vi "Localization Demo.vi"() -> ()   [LabVIEW 2019]
uses:
  SubVIs/RegisterVI.vi
  <vilib>/Platform/browser.llb/Open URL in Default Browser (string).vi
panel:
  in  "Button with Multiple Strings":bool
  out "Current Date and Time":string caption="Current Date or Time"
  in  "Date and Time":u16(ring) items=["Show Localized Time", "Show Localized Date"]
  in  "Show Dialog":bool caption="Show Localized Dialog"
  in  "Language ListBox":i32(listbox) caption="Language"
  out "Data.Display":dbl(graph) caption="Incoming Data"
  out "Error":bool
  in  "CustomControl.Increment":bool caption="Increment"
  out "Count":dbl
  in  "Exit":bool
  # "Instructions:\n1. Run this VI\n2. Toggle the language selector to show the language you would like to show\n3. Observe that the text on the VI changes language\n4. Push the button that says \"Show Localized Dialog.\" This will call Localize Phrase to show a dialog with a localized phrase.\n5. Check out the github page for more documentation and details\nhttps://github.com/JKISoftware/JKI-Simple-Localization"
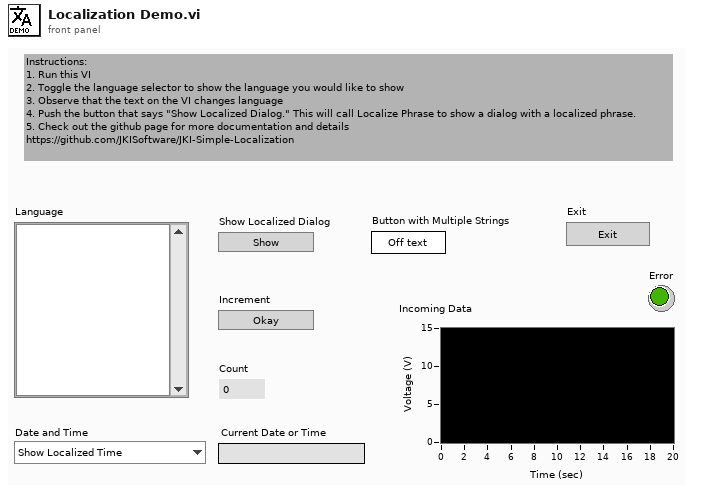
[diagram p1: front panel]
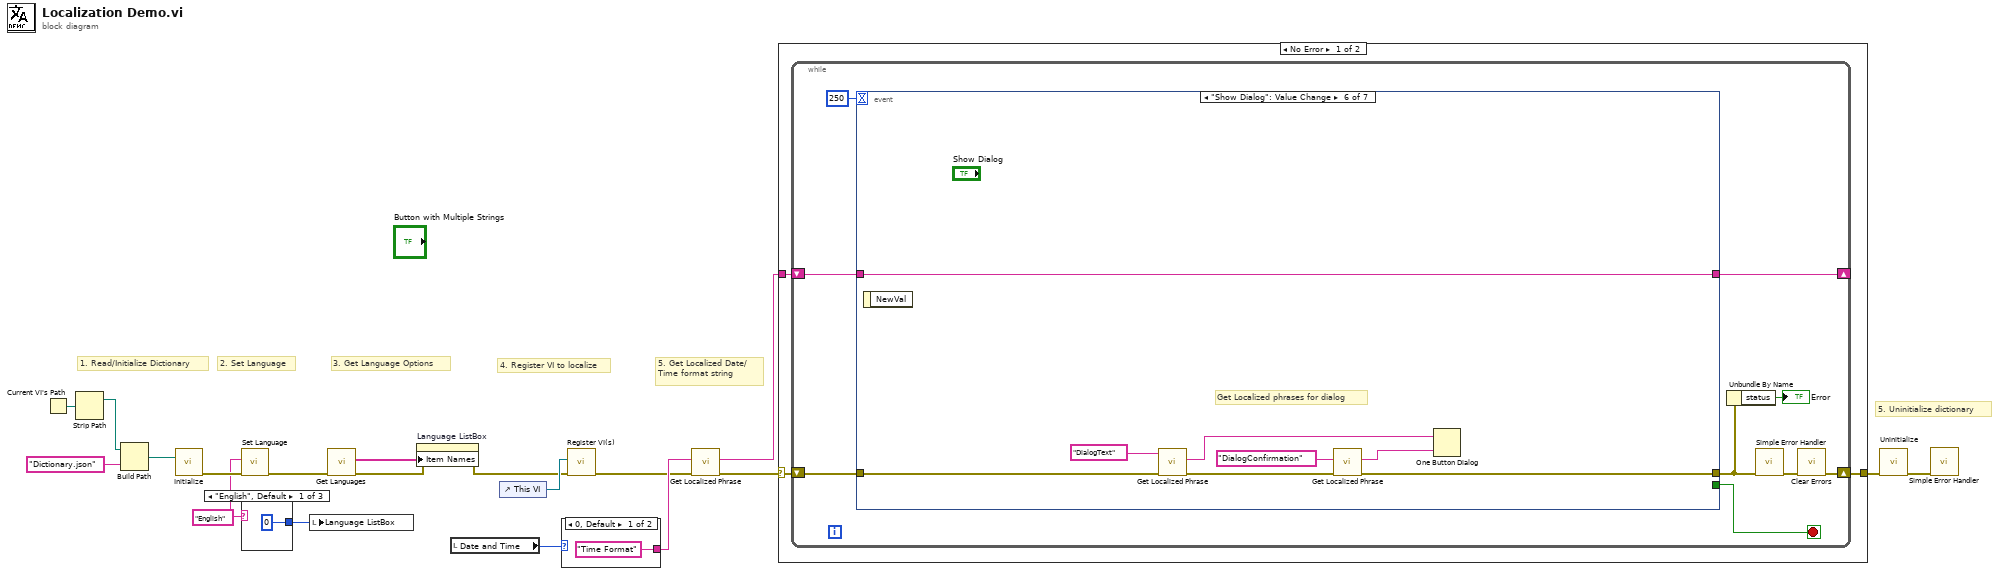
[diagram p0: block diagram]
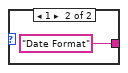
[diagram p2: hidden frame]
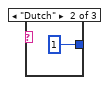
[diagram p3: hidden frame]
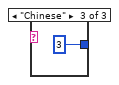
[diagram p4: hidden frame]
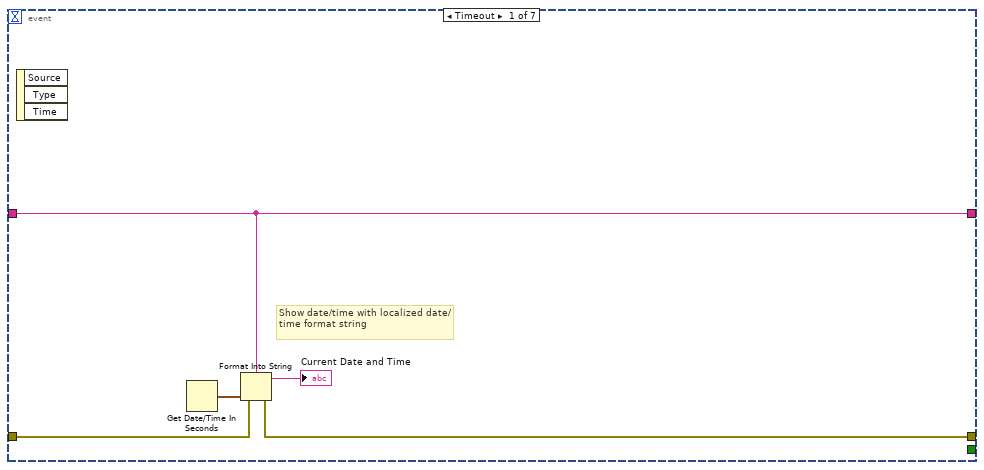
[diagram p5: hidden frame]
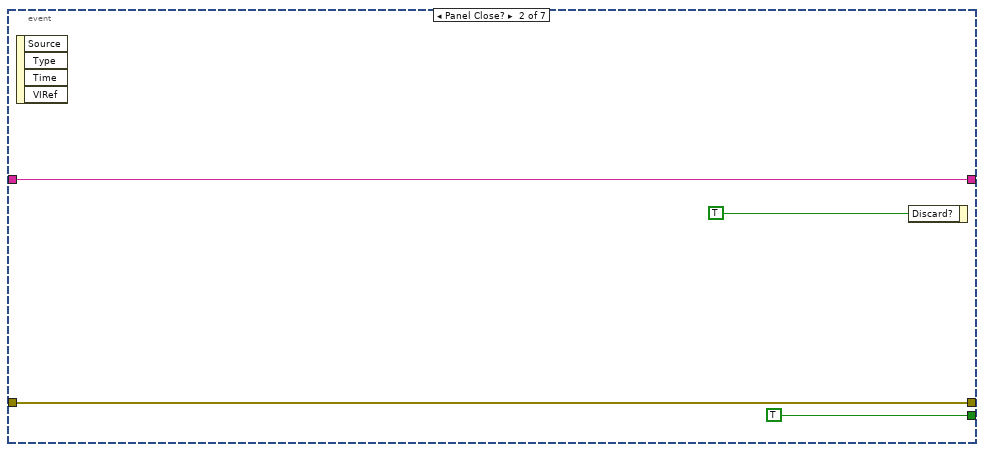
[diagram p6: hidden frame]
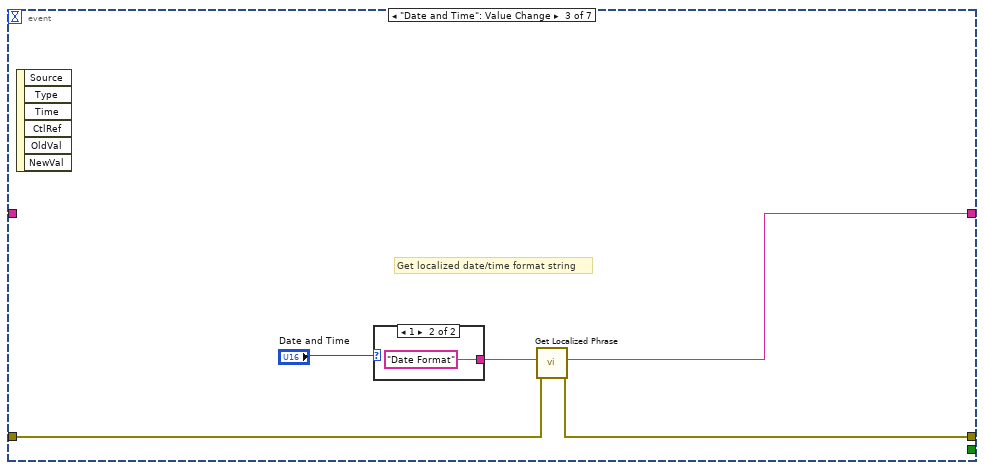
[diagram p7: hidden frame]
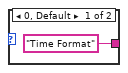
[diagram p8: hidden frame]
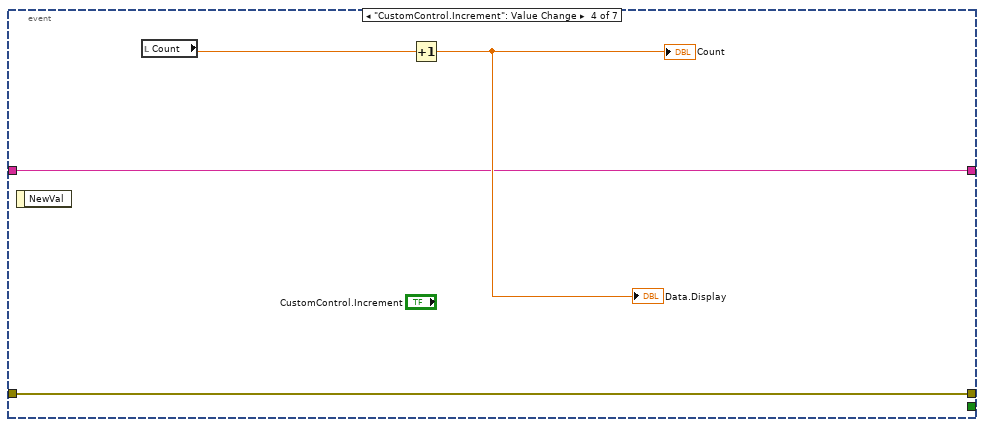
[diagram p9: hidden frame]
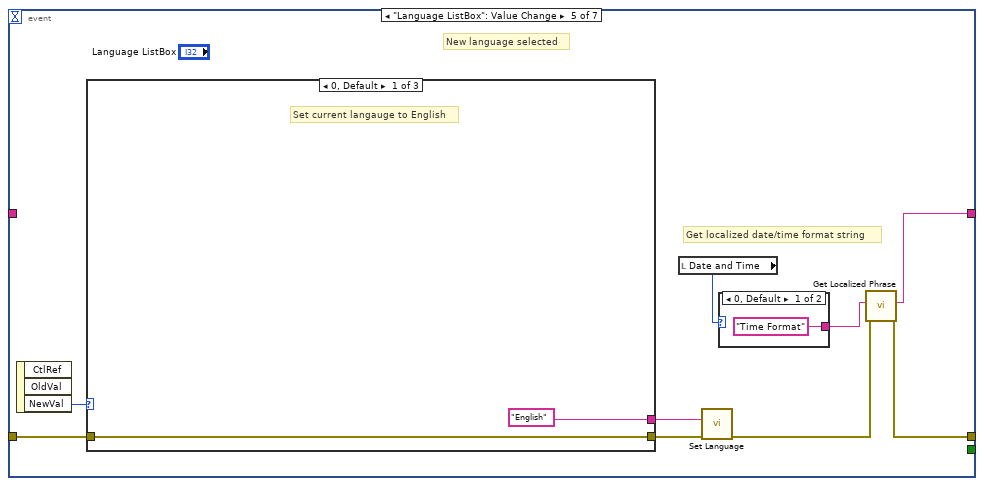
[diagram p10: hidden frame]
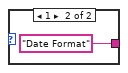
[diagram p11: hidden frame]
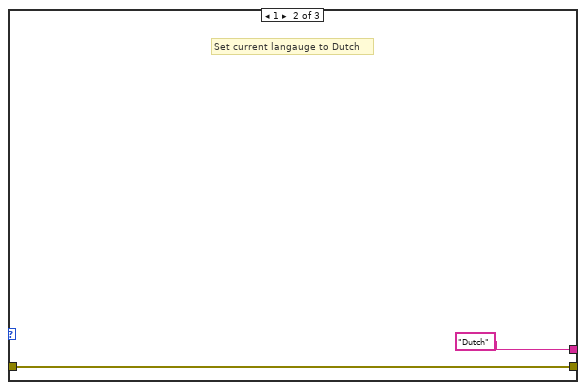
[diagram p12: hidden frame]
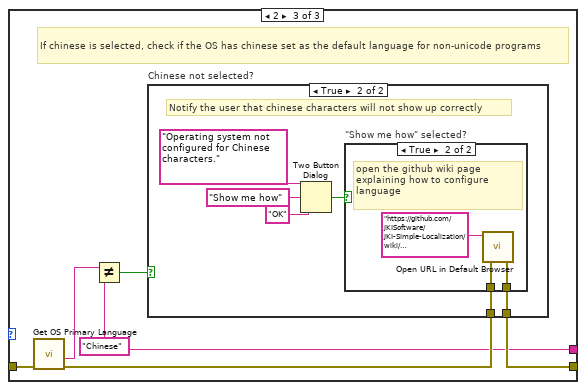
[diagram p13: hidden frame]
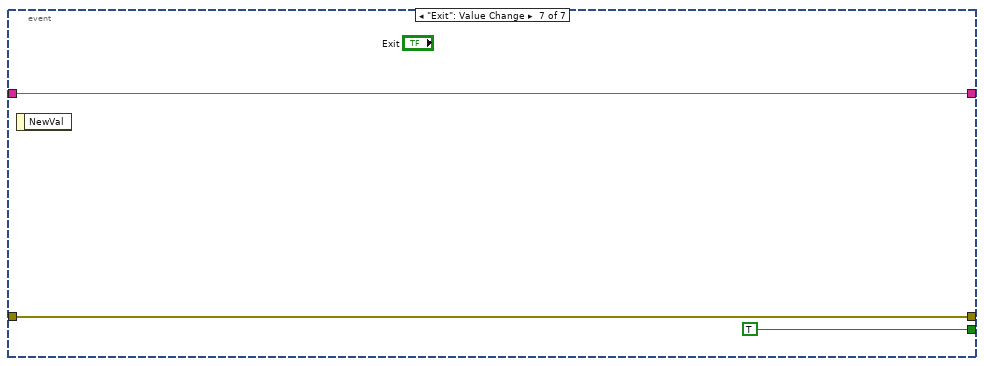
[diagram p16: hidden frame]
diagram:
  w7 = "English" ("Target Language (current lang)")
  # "5. Uninitialize dictionary"
  # "5. Get Localized Date/Time format string"
  # "4. Register VI to localize"
  # "3. Get Language Options"
  # "2. Set Language"
  # "1. Read/Initialize Dictionary"
  n1 = Current VI's Path() -> (path=w11:path)
  n2 = Strip Path(path=w11) -> (stripped path=w10:path)  [unwired: 1 out]
  n3 = Build Path(base path=w10, name or relative path="Dictionary.json") -> (appended path=w19:path)
  n4 = call "Initialize.vi"("Dictionary File Path"=w19) -> ("error out"=w9:errorcluster)  [unwired: 9 in, 5 out]
  n5 = call "Set Language.vi"("error in"=w9, "Target Language (current lang)"=w7) -> ("error out"=w8:errorcluster)  [unwired: 8 in, 1 out]
  n6 = case shown="\"English\", Default" w7 {
    tunnel: [0 ("Language ListBox") 1 ("Language ListBox") 3 ("Language ListBox")] -> w13
    frame "English", Default {
    }
    frame "Dutch" {
    }
    frame "Chinese" {
    }
  }
  n7 = local write "Language ListBox"(w13) -> ()
  n8 = call "Get Languages.vi"("error in"=w8) -> ("error out"=w16:errorcluster, "Languages"=w17:string[])  [unwired: 9 in]
  n9 = property on="Language ListBox" class="LstBox (strict)"(error in=w16, "Item Names"=w17) -> (error out=w14:errorcluster)  [unwired: 1 in, 1 out]
  n10 = local read "Date and Time"() -> (w2:u16)
  n11 = control-ref of="This VI"() -> (w18:refnum<vi>)
  n12 = case shown="0, Default" w2 {
    tunnel: ["Time Format" ("Key") "Date Format" ("Key")] -> w5
    frame 0, Default {
    }
    frame 1 {
    }
  }
  n13 = call-poly "Register VI(s).vi"("error in"=w14, "VI Ref"=w18) -> ("error out"=w4:errorcluster)  [unwired: 8 in, 1 out]
  n14 = call "Get Localized Phrase.vi"("error in"=w4, "Key"=w5) -> ("error out"=w3:errorcluster, "Translated Phrase"=w1:string)  [unwired: 8 in]
  n15 = case shown="No Error" w3 {
    selector: w3 -> [w26 w100]
    tunnel: [w27 w100] -> w15
    tunnel: w1 -> [w25 _]
    frame No Error {
      n16 = while {
        shift-right: [w33] -> w27
        shift-left: w26 -> [w35]
        shift-right: [w28] -> _
        shift-left: w25 -> [w29]
        stop <- w36 stop-if-true
        n17 = event shown="[5] \"Show Dialog\": Value Change" {
          selector: _ -> [_ _ _ _ _ _ _]
          dyn-events: _ -> [_ _ _ _ _ _ _]
          timeout: 250 -> [_ _ _ _ _ _ _]
          tunnel: [_ TRUE _ _ _ _ TRUE ("Exit")] -> w36
          tunnel: [w39 w45 w47 w54 w58 w92 w99] -> w31
          tunnel: w35 -> [w40 w45 w48 w54 w63 w96 w99]
          tunnel: w29 -> [w37 w42 _ w53 _ w89 w97]
          tunnel: [w37 w42 w46 w53 w60 w89 w97] -> w28
          event Timeout {
            # "Show date/time with localized date/time format string"
            n18 = event-data() -> ()  [unwired: 1 in, 3 out]
            n19 = Get Date/Time In Seconds() -> (seconds since 1Jan1904=w41:timestamp)
            n20 = Format Into String(format string=w37, error in=w40, w41) -> (resulting string=→"Current Date and Time":string, error out=w39:errorcluster)  [unwired: 1 in]
          }
          event Panel Close? {
            n21 = event-data() -> ()  [unwired: 1 in, 4 out]
            n22 = event-data("Discard?"=TRUE) -> ()  [unwired: 1 in, 1 out]
          }
          event "Date and Time": Value Change {
            # "Get localized date/time format string"
            n23 = event-data() -> ()  [unwired: 1 in, 6 out]
            n24 = case shown="1" "Date and Time" {
              tunnel: ["Time Format" ("Key") "Date Format" ("Key")] -> w50
              frame 0, Default {
              }
              frame 1 {
              }
            }
            n25 = call "Get Localized Phrase.vi"("error in"=w48, "Key"=w50) -> ("error out"=w47:errorcluster, "Translated Phrase"=w46:string)  [unwired: 8 in]
          }
          event "CustomControl.Increment": Value Change {
            n26 = event-data() -> ()  [unwired: 1 in, 1 out]
            n27 = local read "Count"() -> (w56:dbl)
            n28 = Increment(x=w56) -> (x+1=→"Count" →"Data.Display":dbl)
          }
          event "Language ListBox": Value Change {
            # "Get localized date/time format string"
            # "New language selected"
            n29 = event-data() -> ("NewVal"=w65:i32)  [unwired: 1 in, 2 out]
            n30 = case shown="0, Default" w65 {
              tunnel: ["English" ("name or relative path") "Dutch" ("name or relative path") w72] -> w64
              tunnel: w63 -> [w68 w70 w77]
              tunnel: [w68 w70 w73] -> w62
              frame 0, Default {
                # "Set current langauge to English"
              }
              frame 1 {
                # "Set current langauge to Dutch"
              }
              frame 2 {
                w72 = "Chinese" ("name or relative path")
                # "If chinese is selected, check if the OS has chinese set as the default language for non-unicode programs"
                n31 = call "Get OS Primary Language.vi"("error in"=w77) -> ("error out"=w74:errorcluster, "OS Primary Language"=w76:string)  [unwired: 9 in]
                n32 = Not Equal?(x=w76, y=w72) -> (x != y?=w75:bool)
                n33 = case "Chinese not selected?" shown="True" w75 {
                  tunnel: w74 -> [w78 w81]
                  tunnel: [w78 w80] -> w73
                  frame False {
                    # "Chinese characters will show up correctly"
                  }
                  frame True {
                    # "Notify the user that chinese characters will not show up correctly"
                    n34 = Two Button Dialog(message="Operating system not configured for Chinese characters.", 1:"OK" ("F button name (\"Cancel\")"), 2:"Show me how" ("T button name (\"OK\")")) -> (T button?=w82:bool)
                    n35 = case "\"Show me how\" selected?" shown="True" w82 {
                      tunnel: w81 -> [w85 w87]
                      tunnel: [w85 w86] -> w80
                      frame False {
                      }
                      frame True {
                        # "open the github wiki page explaining how to configure language"
                        n36 = call-poly <vilib>:"Open URL in Default Browser.vi"("error in (no error)"=w87, "URL"="https://github.com/JKISoftware/JKI-Simple-Localization/wiki/Configuring-Windows-Language-(System-Locale)") -> ("error out"=w86:errorcluster)  [unwired: 4 in, 1 out]
                      }
                    }
                  }
                }
              }
            }
            n37 = local read "Date and Time"() -> (w57:u16)
            n38 = call "Set Language.vi"("error in"=w62, "Target Language (current lang)"=w64) -> ("error out"=w59:errorcluster)  [unwired: 8 in, 1 out]
            n39 = case shown="0, Default" w57 {
              tunnel: ["Time Format" ("Key") "Date Format" ("Key")] -> w61
              frame 0, Default {
              }
              frame 1 {
              }
            }
            n40 = call "Get Localized Phrase.vi"("error in"=w59, "Key"=w61) -> ("error out"=w58:errorcluster, "Translated Phrase"=w60:string)  [unwired: 8 in]
          }
          event "Show Dialog": Value Change {
            # "Get Localized phrases for dialog"
            n41 = event-data() -> ()  [unwired: 1 in, 1 out]
            n42 = call "Get Localized Phrase.vi"("error in"=w96, "Key"="DialogText") -> ("error out"=w93:errorcluster, "Translated Phrase"=w94:string)  [unwired: 8 in]
            n43 = call "Get Localized Phrase.vi"("error in"=w93, "Key"="DialogConfirmation") -> ("error out"=w92:errorcluster, "Translated Phrase"=w90:string)  [unwired: 8 in]
            n44 = One Button Dialog(message=w94, button name ("OK")=w90) -> ()  [unwired: 1 out]
          }
          event "Exit": Value Change {
            n45 = event-data() -> ()  [unwired: 1 in, 1 out]
          }
        }
        n46 = Unbundle By Name(w31) -> ("status"=→"Error":bool)
        n47 = call <vilib>:"Simple Error Handler.vi"("error in (no error)"=w31) -> ("error out"=w32:errorcluster)  [unwired: 4 in, 4 out]
        n48 = call <vilib>:"Clear Errors.vi"("error in (no error)"=w32) -> ("error out"=w33:errorcluster)  [unwired: 5 in, 1 out]
      }
    }
    frame Error {
    }
  }
  n49 = call "Uninitialize.vi"("error in"=w15) -> ("error out"=w12:errorcluster)  [unwired: 10 in]
  n50 = call <vilib>:"Simple Error Handler.vi"("error in (no error)"=w12) -> ()  [unwired: 4 in, 5 out]
